vi "BT_to_neon.vi"() -> ()   [LabVIEW 2016]
uses:
  Typedef/Type_of_message_to_MCU.ctl
  Typedef/MCU_addresses.ctl
  Typedef/Serial_config_cluster.ctl
  <vilib>/Instr/_visa.llb/VISA Configure Serial Port (Instr).vi
panel:
  out "error out":errorcluster
  in  "Cluster 2":T1={"Termination Character"=10, "End Read on"=TRUE, "VISA resource name"="COM1", "baud rate"=9600, "data bits"=8, "parity"=enum."None", "stop bits"=10, "flow control"=0, "XON"=enum."DC1", "XOFF"=enum."DC3", "End Write on"=FALSE} {"Termination Character" format="%.0x"; "flow control" items=["None"=0, "XON/XOFF"=1, "RTS/CTS"=2, "DTR/DSR"=4]; "data bits" min=5 max=8 step=1; "stop bits" items=["1.0"=10, "1.5"=15, "2.0"=20]; "baud rate" items=["75"=75, "110"=110, "134"=134, "150"=150, "300"=300, "600"=600, "1200"=1200, "1800"=1800, "2400"=2400, "4800"=4800, "7200"=7200, "9600"=9600, "14400"=14400, "19200"=19200, "28800"=28800, "38400"=38400, "56000"=56000, "57600"=57600, "115200"=115200, "128000"=128000, "230400"=230400]}
  in  "Stop\n 2":bool
  in  "Read Count 2":u32=1000
  out "String 2":string
  out "Extracted Numbers 2":dbl[](array[numeric]) format="%#.6g"
  in  "Save 2":bool=TRUE
  out "Byte array has been sent 2":u8[](array[numeric])
  in  "MCU Address to be sent 2":T2
  in  "Payload  Byte to be sent 2":u8[](array[numeric])
  in  "Types of Data 2":T3
  in  "Read 2":bool=TRUE
  out "Bytes at Serial Port 2":u32
  out "error out 3":errorcluster
  in  "MAIN STOP 2":bool
  out "MAIN STOP OUT 2":bool
  in  "sEND":bool
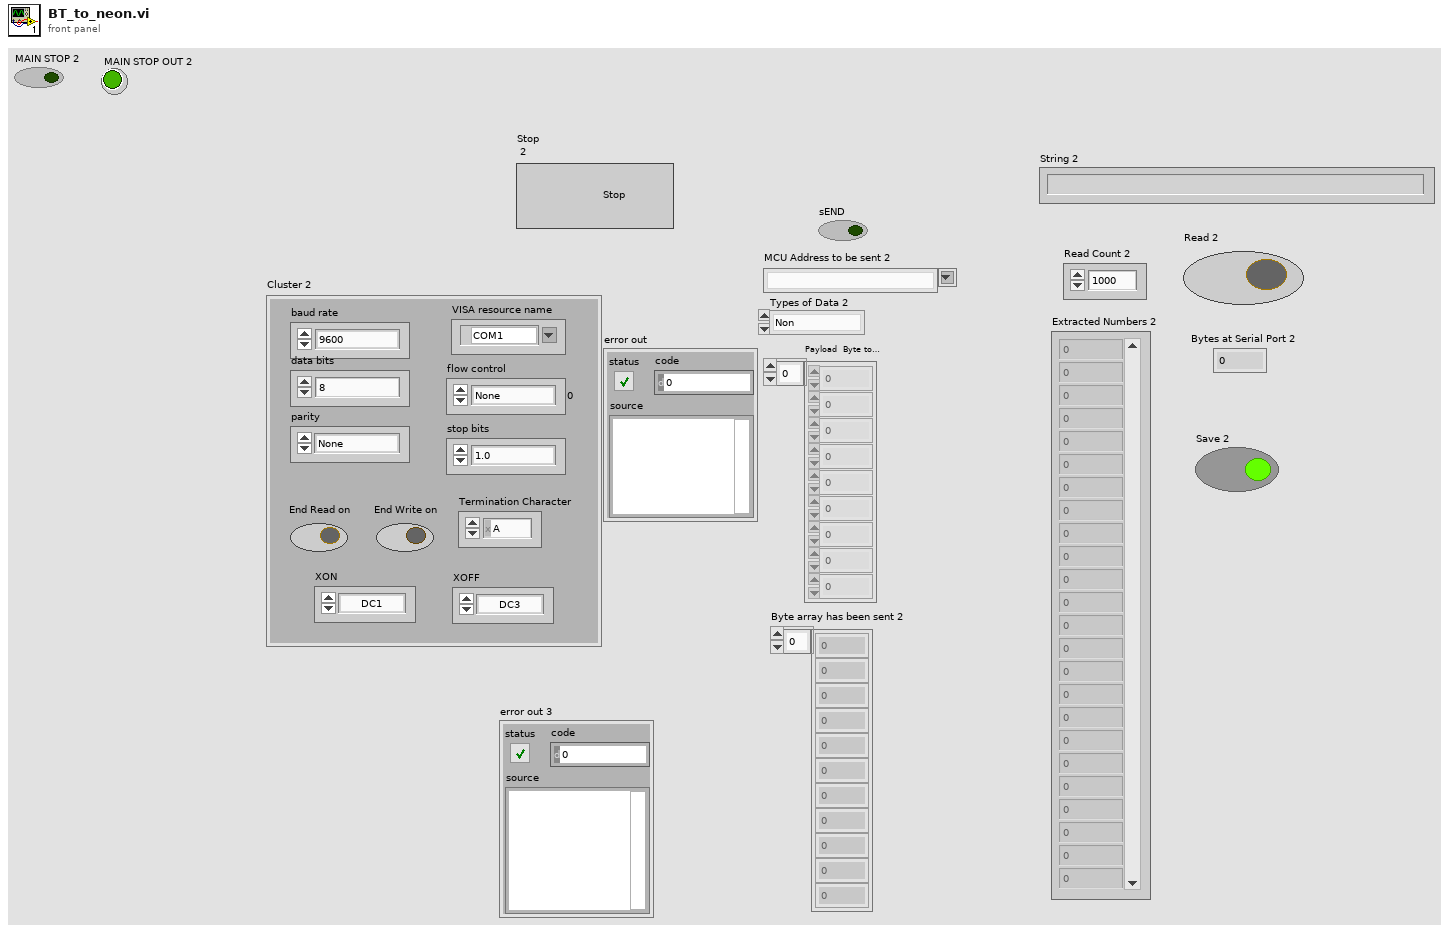
[diagram p1: front panel]
types:
  T1 = typedef "Serial_config_cluster.ctl" = cluster{"Termination Character":u8, "End Read on":bool, "VISA resource name":refnum<visa-resource-name>, "baud rate":u32, "data bits":u16, "parity":enum16{"None", "Odd", "Even", "Mark", "Space"}, "stop bits":u16, "flow control":u16, "XON":enum16{"NUL", "SOH", "STX", "ETX", "EOT", "ENQ", "ACK", "BEL", "BS", "HT", "LF", "VT", "FF", "CR", "SO", "SI", "DLE", "DC1", "DC2", "DC3", "DC4", "NAK", "SYN", "ETB", "CAN", "EM", "SUB", "ESC", "FS", "GS", "RS", "US", "SP", "!", "\"", "#", "$", "%", "&", "'", "(", ")", "*", "+", ",", "- (-)", ".", "/", "0", "1", "2", "3", "4", "5", "6", "7", "8", "9", ":", ";", "<", "=", ">", "?", "@", "A", "B", "C", "D", "E", "F", "G", "H", "I", "J", "K", "L", "M", "N", "O", "P", "Q", "R", "S", "T", "U", "V", "W", "X", "Y", "Z", "[", "\\", "]", "^", "_", "`", "a", "b", "c", "d", "e", "f", "g", "h", "i", "j", "k", "l", "m", "n", "o", "p", "q", "r", "s", "t", "u", "v", "w", "x", "y", "z", "{", "|", "}", "~"}, "XOFF":enum16{"NUL", "SOH", "STX", "ETX", "EOT", "ENQ", "ACK", "BEL", "BS", "HT", "LF", "VT", "FF", "CR", "SO", "SI", "DLE", "DC1", "DC2", "DC3", "DC4", "NAK", "SYN", "ETB", "CAN", "EM", "SUB", "ESC", "FS", "GS", "RS", "US", "SP", "!", "\"", "#", "$", "%", "&", "'", "(", ")", "*", "+", ",", "- (-)", ".", "/", "0", "1", "2", "3", "4", "5", "6", "7", "8", "9", ":", ";", "<", "=", ">", "?", "@", "A", "B", "C", "D", "E", "F", "G", "H", "I", "J", "K", "L", "M", "N", "O", "P", "Q", "R", "S", "T", "U", "V", "W", "X", "Y", "Z", "[", "\\", "]", "^", "_", "`", "a", "b", "c", "d", "e", "f", "g", "h", "i", "j", "k", "l", "m", "n", "o", "p", "q", "r", "s", "t", "u", "v", "w", "x", "y", "z", "{", "|", "}", "~"}, "End Write on":bool}
  T2 = typedef "MCU_addresses.ctl" = string
  T3 = typedef "Type_of_message_to_MCU.ctl" = enum16{"Non", "Alarm", "Error", "Time and Date", "Status", "Request", "Command"}
  T4 = enum16{"NUL", "SOH", "STX", "ETX", "EOT", "ENQ", "ACK", "BEL", "BS", "HT", "LF", "VT", "FF", "CR", "SO", "SI", "DLE", "DC1", "DC2", "DC3", "DC4", "NAK", "SYN", "ETB", "CAN", "EM", "SUB", "ESC", "FS", "GS", "RS", "US", "SP", "!", "\"", "#", "$", "%", "&", "'", "(", ")", "*", "+", ",", "- (-)", ".", "/", "0", "1", "2", "3", "4", "5", "6", "7", "8", "9", ":", ";", "<", "=", ">", "?", "@", "A", "B", "C", "D", "E", "F", "G", "H", "I", "J", "K", "L", "M", "N", "O", "P", "Q", "R", "S", "T", "U", "V", "W", "X", "Y", "Z", "[", "\\", "]", "^", "_", "`", "a", "b", "c", "d", "e", "f", "g", "h", "i", "j", "k", "l", "m", "n", "o", "p", "q", "r", "s", "t", "u", "v", "w", "x", "y", "z", "{", "|", "}", "~"}
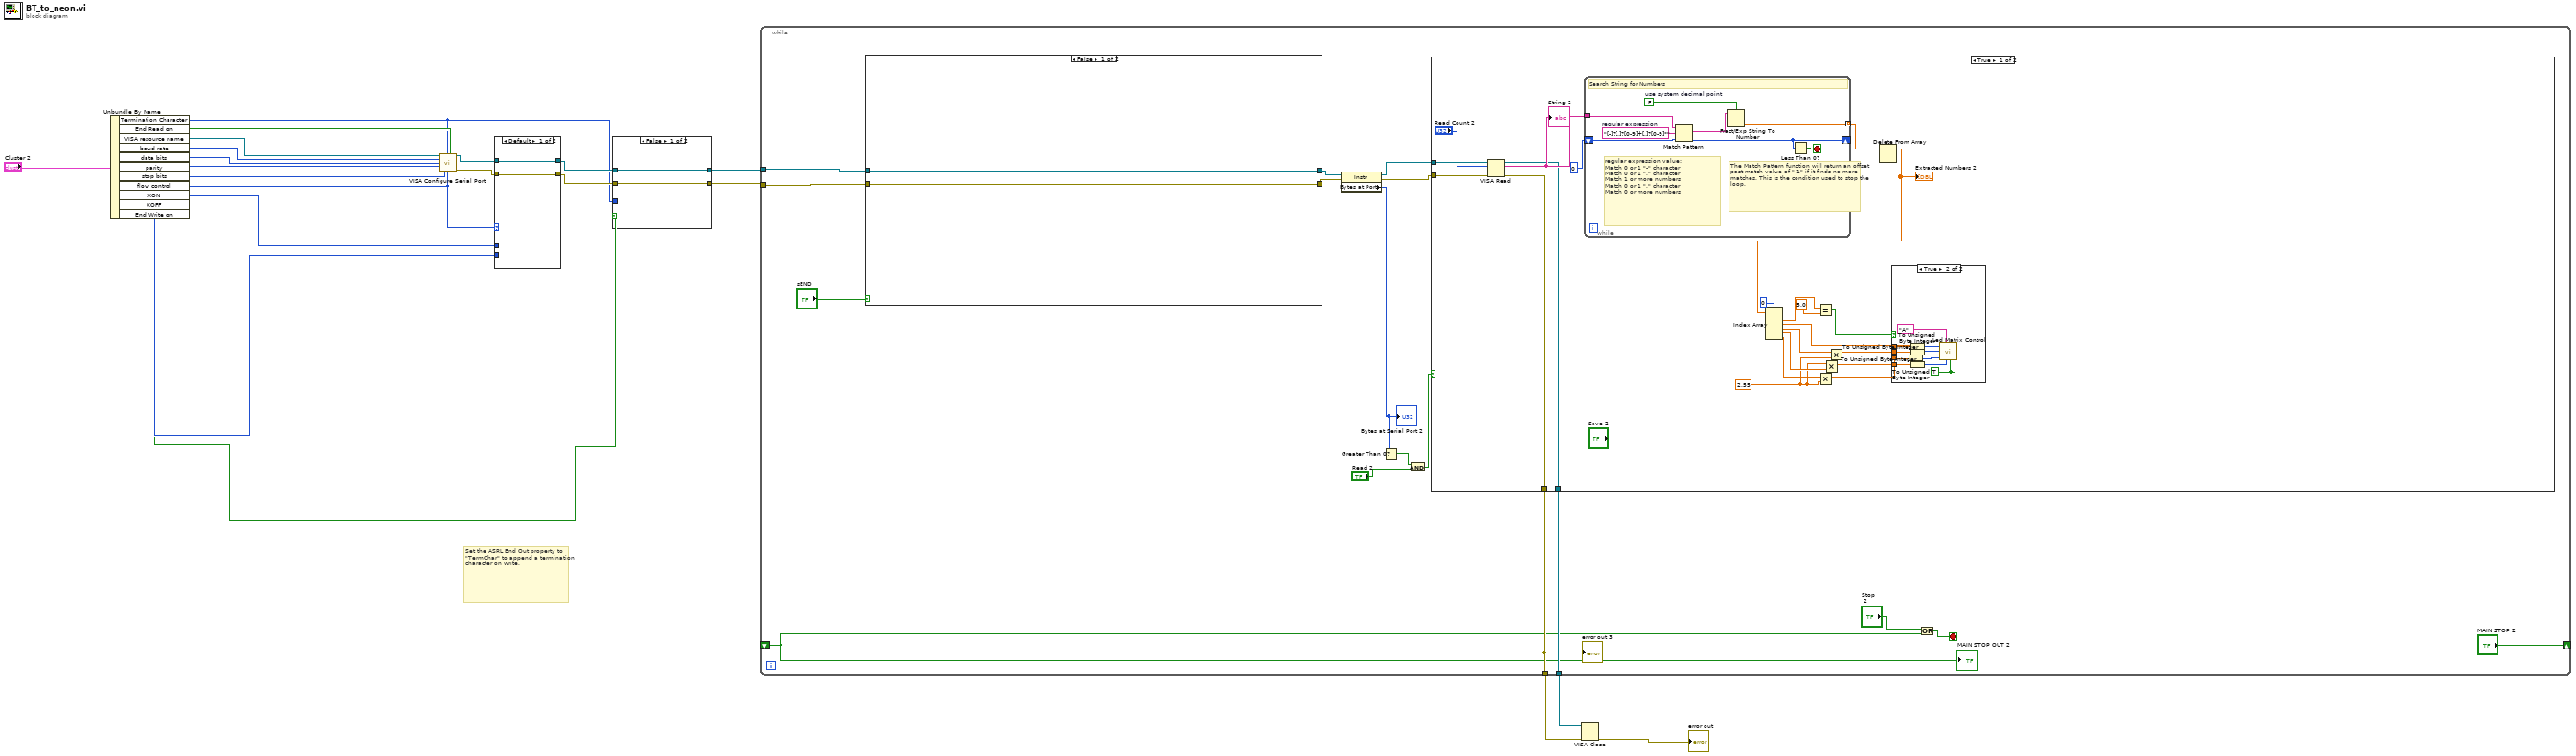
[diagram p0: block diagram]
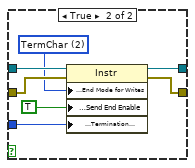
[diagram p2: hidden frame]
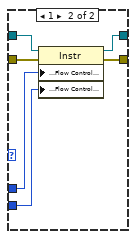
[diagram p3: hidden frame]
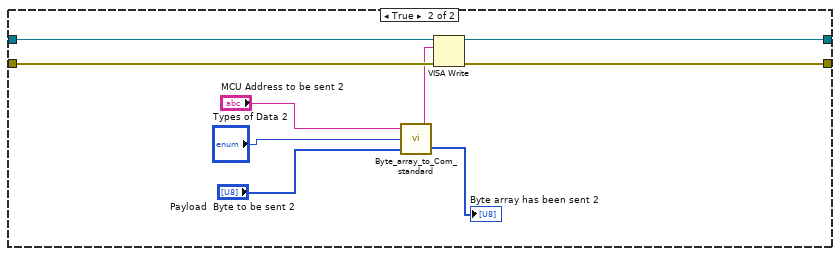
[diagram p4: hidden frame]
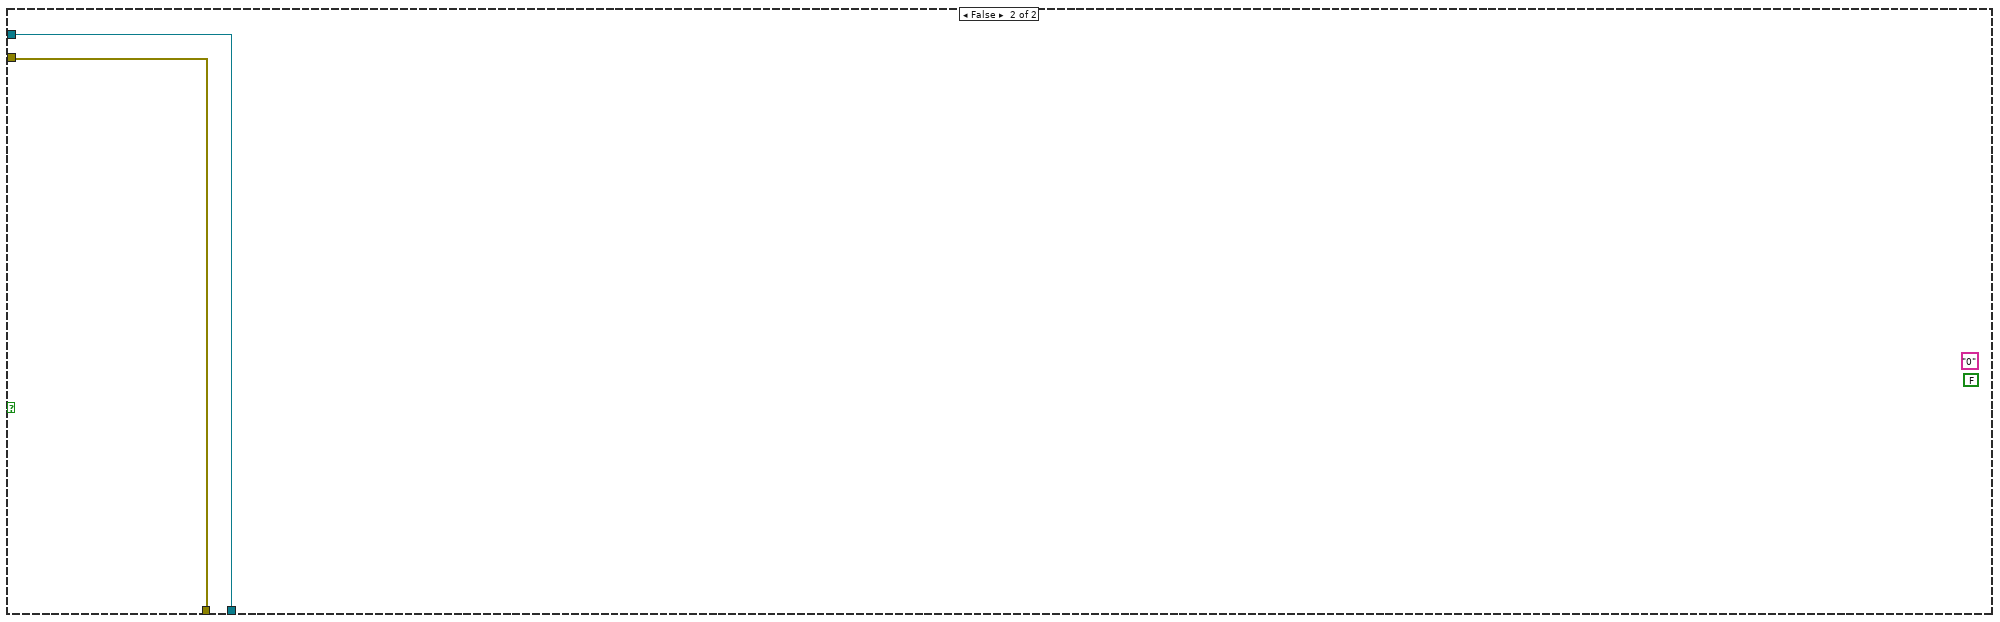
[diagram p6: hidden frame]
diagram:
  # "Set the ASRL End Out property to \"TermChar\" to append a termination character on write."
  n1 = Unbundle By Name("Cluster 2") -> ("Termination Character"=w6:u8, "End Read on"=w15:bool, "VISA resource name"=w16:refnum<visa-resource-name>, "baud rate"=w14:u32, "data bits"=w13:u16, "parity"=w12:enum16{"None", "Odd", "Even", "Mark", "Space"}, "stop bits"=w11:u16, "flow control"=w10:u16, "XON"=w9:T4, "XOFF"=w8:T4, "End Write on"=w7:bool)
  n2 = call-poly "VISA Configure Serial Port"("VISA resource name"=w16, "termination char\n(0xA = '\\n' = LF)"=w6, "Enable Termination\nChar (T)"=w15, "baud rate (9600)"=w14, "data bits (8)"=w13, "parity (0:none)"=w12, "stop bits (10: 1 bit)"=w11, "flow control (0:none)"=w10) -> ("VISA resource name out"=w19:refnum<visa-resource-name>, "error out"=w18:errorcluster)  [unwired: 2 in, 4 out]
  n3 = case shown="Default" w10 {
    tunnel: [w22 w29] -> w20
    tunnel: [w23 w28] -> w21
    tunnel: w18 -> [w22 w27]
    tunnel: w19 -> [w23 w26]
    tunnel: w9 -> [_ w25]
    tunnel: w8 -> [_ w24]
    frame Default {
    }
    frame 1 {
      n4 = property class="Instr"(reference=w26, error in=w27, "Serial Settings:Flow Control XON Character"=w25, "Serial Settings:Flow Control XOFF Character"=w24) -> (reference out=w28:refnum<visa-resource-name>, error out=w29:errorcluster)
    }
  }
  n5 = case shown="False" w7 {
    tunnel: w21 -> [w30 w38]
    tunnel: w20 -> [w31 w37]
    tunnel: [w30 w36] -> w5
    tunnel: [w31 w35] -> w4
    tunnel: w6 -> [_ w33]
    frame False {
    }
    frame True {
      w34 = u16 2 items=["None", "LastBit", "TermChar", "Break"] ("Serial Settings:Serial End Mode for Writes")
      n6 = property class="Instr"(reference=w38, error in=w37, "Serial Settings:End Mode for Writes"=w34, "Message Based Settings:Send End Enable"=TRUE, "Message Based Settings:Termination Character"=w33) -> (reference out=w36:refnum<visa-resource-name>, error out=w35:errorcluster)
    }
  }
  n7 = while {
    tunnel: w5 -> [w48]
    tunnel: w4 -> [w47]
    tunnel: [w45] -> w3
    tunnel: [w44] -> w2
    shift-right: ["MAIN STOP 2"] -> _
    shift-left: _ -> [w40]
    stop <- w42 stop-if-true
    n8 = case shown="False" "sEND" {
      tunnel: w48 -> [w57 w66]
      tunnel: w47 -> [w56 w65]
      tunnel: [w57 w64] -> w49
      tunnel: [w56 w63] -> w51
      frame False {
      }
      frame True {
        n9 = call "Byte_array_to_Com_standard.vi"("Payload  Byte to be sent"="Payload  Byte to be sent 2", "Types of Data"="Types of Data 2", "MCU Address to be sent"="MCU Address to be sent 2") -> ("Byte array has been sent"=→"Byte array has been sent 2":u8[], "Converted Message"=w59:string)
        n10 = VISA Write(VISA resource name=w66, write buffer=w59, error in (no error)=w65) -> (VISA resource name out=w64:refnum<visa-resource-name>, error out=w63:errorcluster)  [unwired: 1 out]
      }
    }
    n11 = property class="Instr"(reference=w49, error in=w51) -> (reference out=w50:refnum<visa-resource-name>, error out=w52:errorcluster, "Bytes at Port"=w53:u32)
    "Bytes at Serial Port 2" <- w53
    n12 = Greater Than 0?(x=w53) -> (x > 0?=w55:bool)
    n13 = And(x=w55, y="Read 2") -> (x .and. y?=w46:bool)
    n14 = case shown="True" w46 {
      tunnel: w50 -> [w87 w107]
      tunnel: w52 -> [w86 w106]
      tunnel: [w82 w107] -> w45
      tunnel: [w81 w106] -> w44
      frame True {
        w67 = 2.55
        n15 = VISA Read(VISA resource name=w87, byte count="Read Count 2", error in (no error)=w86) -> (VISA resource name out=w82:refnum<visa-resource-name>, read buffer=w83:string, error out=w81:errorcluster)  [unwired: 1 out]
        "String 2" <- w83
        n16 = while {
          tunnel: w83 -> [w105]
          shift-left: 0 -> [w103]
          shift-right: [w100] -> _
          tunnel: [w98] -> w79 mode=indexing
          stop <- w104 stop-if-true
          w102 = FALSE  # use system decimal point
          w99 = "[-]?[.]?[0-9]+[.]?[0-9]*"  # regular expression
          # "The Match Pattern function will return an offset past match value of \"-1\" if it finds no more matches. This is the condition used to stop the loop."
          # "regular expression value:\nMatch 0 or 1 \"-\" character\nMatch 0 or 1 \".\" character\nMatch 1 or more numbers\nMatch 0 or 1 \".\" character\nMatch 0 or more numbers"
          # "Search String for Numbers"
          n17 = Match Pattern(string=w105, regular expression=w99, offset (0)=w103) -> (match substring=w101:string, offset past match=w100:i32)  [unwired: 2 out]
          n18 = Fract/Exp String To Number(use system decimal point (T)=w102, string=w101) -> (number=w98:dbl)  [unwired: 2 in, 1 out]
          n19 = Less Than 0?(x=w100) -> (x < 0?=w104:bool)
        }
        n20 = Delete From Array(array=w79) -> (array with subset deleted=w71:dbl[])  [unwired: 2 in, 1 out]
        "Extracted Numbers 2" <- w71
        n21 = Index Array(array=w71, index #1=0 ("length")) -> (element #1=w77:dbl, element #2=w75:dbl, element #3=w74:dbl, element #4=w73:dbl, element #5=w72:dbl)  [unwired: 4 in]
        n22 = Equal?(x=w77, y=5.0) -> (x = y?=w76:bool)
        n23 = Multiply(x=w72, y=w67) -> (x*y=w68:dbl)
        n24 = Multiply(x=w67, y=w73) -> (x*y=w69:dbl)
        n25 = Multiply(x=w74, y=w67) -> (x*y=w70:dbl)
        n26 = case shown="True" w76 {
          tunnel: w75 -> [_ w96]
          tunnel: w70 -> [_ w95]
          tunnel: w69 -> [_ w94]
          tunnel: w68 -> [_ w93]
          frame False {
          }
          frame True {
            w88 = TRUE ("Close Tab")
            n27 = To Unsigned Byte Integer(number=w94) -> (unsigned 8bit integer=w90:u8)
            n28 = To Unsigned Byte Integer(number=w96) -> (unsigned 8bit integer=w92:u8)
            n29 = To Unsigned Byte Integer(number=w95) -> (unsigned 8bit integer=w91:u8)
            n30 = To Unsigned Byte Integer(number=w93) -> (unsigned 8bit integer=w89:u8)
            n31 = call "Led Matrix Control.vi"("LED Location"=w92, "MCU addresses"=T2 "A", "Red"=w91, "Green"=w90, "Blue"=w89, "Send To MCU"=w88, "Close Tab"=w88) -> ()  [unwired: 2 in, 1 out]
          }
        }
      }
      frame False {
        (unwired) FALSE ("Send/notsend")
        (unwired) "0" ("Converted Message")
      }
    }
    "error out 3" <- w44
    n32 = Or(x="Stop\n 2", y=w40) -> (x .or. y?=w42:bool)
    "MAIN STOP OUT 2" <- w40
  }
  n33 = VISA Close(VISA resource name=w3, error in (no error)=w2) -> (error out=→"error out":errorcluster)
